vi "modeSel.vi"(10 "Buttons[7]":bool, 11 "Buttons[7] 2":bool) -> (3 "Numeric":i32)   [LabVIEW 2014]
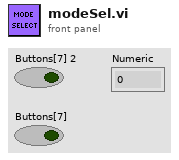
[diagram p1: front panel]
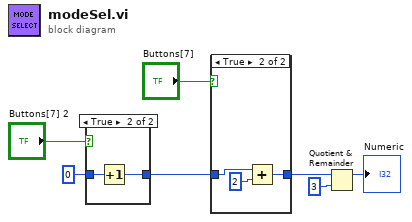
[diagram p0: block diagram]
diagram:
  n1 = case shown="True" "Buttons[7] 2" {
    tunnel: 0 -> [w8 w10]
    tunnel: [w8 w9] -> w3
    frame False {
    }
    frame True {
      n2 = Increment(x=w10) -> (x+1=w9:i32)
    }
  }
  n3 = case shown="True" "Buttons[7]" {
    tunnel: w3 -> [w11 w14]
    tunnel: [w11 w12] -> w5
    frame False {
    }
    frame True {
      n4 = Add(x=w14, y=2) -> (x+y=w12:i32)
    }
  }
  n5 = Quotient & Remainder(x=w5, y=3) -> (x-y*floor(x/y)=→"Numeric":i32)  [unwired: 1 out]
